vi "FollowALine2.vi"   [LabVIEW 2016, in "LEGO-PMR.lvrbt"]
uses:
  LEGO-PMR.lvrbt
  <vilib>/NXT/Block Support/NXT_InputPort.ctl
  <vilib>/NXT/Block Support/NXT_OutputPort.ctl
  <vilib>/NXT/Dual Mode Library/Sensors/EV3_Color_Color.vi
  <vilib>/NXT/Dual Mode Library/Waits/Wait_Num(msec).vi
  <vilib>/NXT/NXTIO Xnodes/NXTIONodeSubVIs/NXTMoveMotors.vi
  <vilib>/NXT/NXTIO Xnodes/NXTIONodeSubVIs/NXTStopMotors.vi
  <vilib>/NXT/NXTIO Xnodes/AddressXNode/NXTIOAddress.xnode
  <vilib>/NXT/NXTIO Xnodes/NXTIOXNode/NXTIO.xnode
  <vilib>/NXT/Subs/LVHSConnector.ctl
  <vilib>/NXT/LegoClasses/BrickReference/BrickReference.lvclass
types:
  T1 = typedef "NXT_InputPort.ctl" = u32
  T2 = typedef "ColorSensorColors.ctl" = enum16{"No Color", "Black", "Blue", "Green", "Yellow", "Red", "White", "Brown"}
  T3 = typedef "LVHSConnector.ctl" = refnum<class "BrickReference.lvclass">
  T4 = typedef "NXT_OutputPort.ctl" = u8
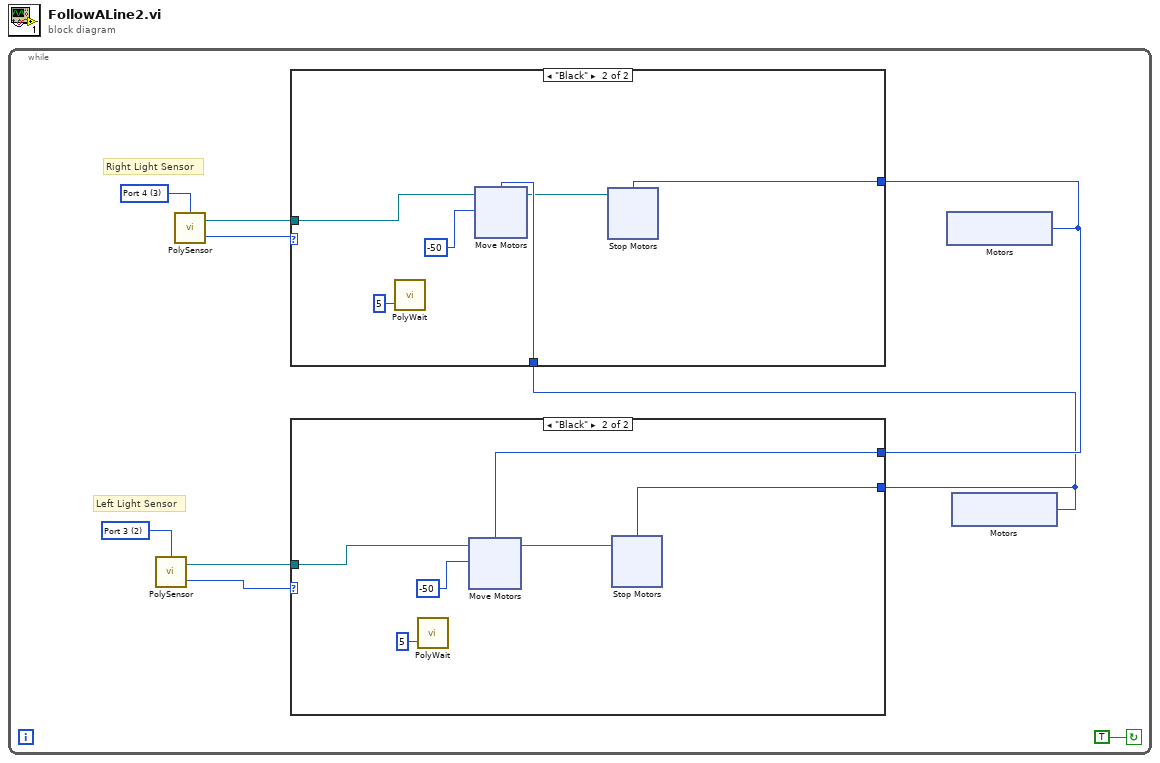
[diagram p0: block diagram]
diagram:
  n1 = while {
    stop <- TRUE continue-if-true
    w6 = T1 3 items=["Port 1", "Port 2", "Port 3", "Port 4"] ("Port (Port 1)")
    w7 = T1 2 items=["Port 1", "Port 2", "Port 3", "Port 4"] ("Port (Port 1)")
    # "Left Light Sensor"
    # "Right Light Sensor"
    n2 = call-poly <vilib>:"PolySensor.vi"("Port (Port 1)"=w7) -> ("Detected Color"=w8:T2, "NXT/EV3"=w3:T3)  [unwired: 2 in]
    n3 = call-poly <vilib>:"PolySensor.vi"("Port (Port 1)"=w6) -> ("Detected Color"=w9:T2, "NXT/EV3"=w2:T3)  [unwired: 2 in]
    n4 = xnode "Motors"() -> ("Motor"=w5:T4)
    n5 = xnode "Motors"() -> ("Motor"=w4:T4)
    n6 = case shown="\"Black\"" w9 {
      tunnel: w5 -> [_ w34]
      tunnel: w4 -> [_ w33]
      tunnel: w2 -> [_ w32]
      frame "No Color", Default {
      }
      frame "Black" {
        n7 = call-poly <vilib>:"PolyWait.vi"("Time (100 msec)"=u32 5) -> ()  [unwired: 3 in, 1 out]
        n8 = xnode "Move Motors"("Power/Speed 1"=-50, "Motors"=w33, "NXT/EV3"=w32) -> ("NXT/EV3"=w31:T3)
        n9 = xnode "Stop Motors"("Motors"=w34, "NXT/EV3"=w31) -> ()  [unwired: 1 out]
      }
    }
    n10 = case shown="\"Black\"" w8 {
      tunnel: w5 -> [_ w16]
      tunnel: w4 -> [_ w15]
      tunnel: w3 -> [_ w14]
      frame "No Color", Default {
      }
      frame "Black" {
        n11 = call-poly <vilib>:"PolyWait.vi"("Time (100 msec)"=u32 5) -> ()  [unwired: 3 in, 1 out]
        n12 = xnode "Move Motors"("Power/Speed 1"=-50, "Motors"=w16, "NXT/EV3"=w14) -> ("NXT/EV3"=w13:T3)
        n13 = xnode "Stop Motors"("Motors"=w15, "NXT/EV3"=w13) -> ()  [unwired: 1 out]
      }
    }
  }
